vi "경로.vi"() -> ()   [LabVIEW 2014]
panel:
  out "에러 출력":errorcluster
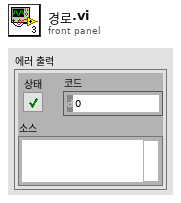
[diagram p1: front panel]
types:
  T1 = enum16{"open", "replace", "create", "open or create", "replace or create", "replace or create with confirmation"}
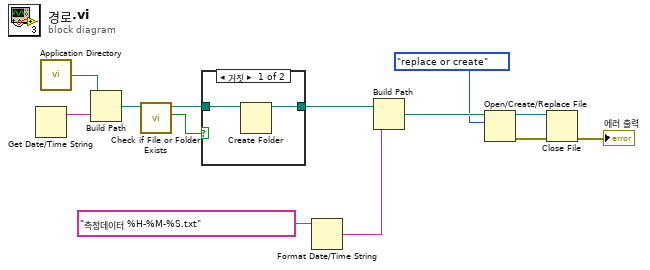
[diagram p0: block diagram]
diagram:
  n1 = Get Date/Time String() -> (date string=w1:string)  [unwired: 3 in, 1 out]
  n2 = call <vilib>:"Application Directory.vi"() -> ("Application Directory"=w11:path)
  n3 = Build Path(base path=w11, name or relative path=w1) -> (appended path=w10:path)
  n4 = call <vilib>:"Check if File or Folder Exists.vi"("path"=w10) -> ("file or folder exists?"=w9:bool, "dup path"=w8:path)  [unwired: 8 in, 1 out]
  n5 = case shown="거짓" w9 {
    tunnel: w8 -> [w15 w16]
    tunnel: [w14 w16] -> w7
    frame False {
      n6 = Create Folder(path (use dialog)=w15) -> (created path=w14:path)  [unwired: 2 in, 2 out]
    }
    frame True {
    }
  }
  n7 = Format Date/Time String(time format string (%c)="측정데이터 %H-%M-%S.txt" ("시간 포맷 문자열 (%c)")) -> (date/time string=w12:string)  [unwired: 2 in]
  n8 = Build Path(base path=w7, name or relative path=w12) -> (appended path=w6:path)
  n9 = Open/Create/Replace File(file path (use dialog)=w6, operation (0:open)=T1."replace or create" ("동작(0:open)")) -> (refnum out=w4:refnum<file>, error out=w3:errorcluster)  [unwired: 4 in, 1 out]
  n10 = Close File(refnum=w4, error in=w3) -> (error out=→"에러 출력":errorcluster)  [unwired: 1 out]
